vi "getViGetNextSample.vi"(8 "error in (no error)":errorcluster, 10 "name":string, 11 "LibReader in":refnum<class "LibReader.lvclass">) -> (0 "error out":errorcluster, 2 "pathViGetNextSample":path, 3 "LibReader out":refnum<class "LibReader.lvclass">)   [LabVIEW 2018, in "LibReader.lvclass"]
doc: "Get the path of get next sample vi."
uses:
  LibReader.lvclass
  LibReader.lvclass/LibReader.ctl
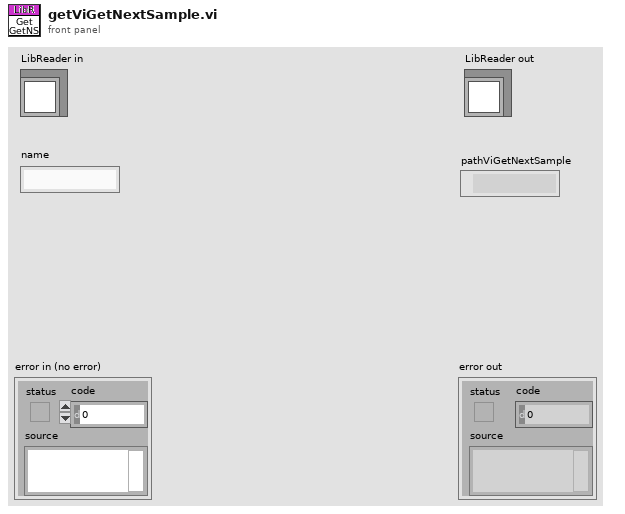
[diagram p1: front panel]
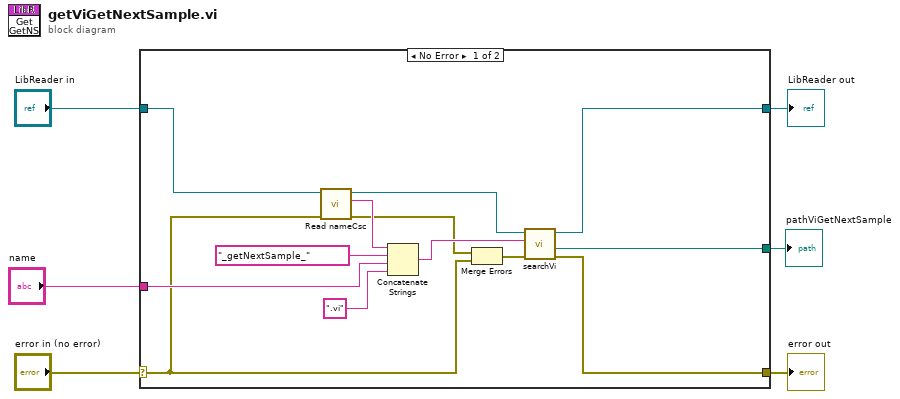
[diagram p0: block diagram]
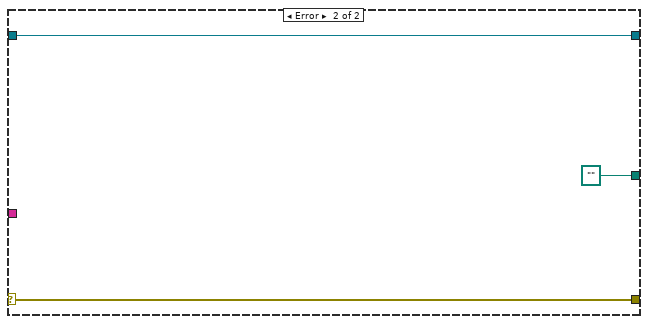
[diagram p2: hidden frame]
diagram:
  n1 = case shown="No Error" "error in (no error)" {
    selector: "error in (no error)" -> [w11 w22]
    tunnel: [w9 w22] -> w5
    tunnel: [w7 w21] -> w3
    tunnel: "LibReader in" -> [w14 w21]
    tunnel: [w19 path "" ("pathVi")] -> w2
    tunnel: "name" -> [w17 _]
    frame No Error {
      n2 = call "Read nameCsc.vi"("error in (no error)"=w11, "LibReader in"=w14) -> ("error out"=w12:errorcluster, "nameCsc"=w13:string, "LibReader out"=w8:refnum<class "LibReader.lvclass">)  [unwired: 7 in]
      n3 = Concatenate Strings(w13, "_getNextSample_" ("regExpr"), w17, ".vi" ("regExpr")) -> (w15:string)
      n4 = Merge Errors(w12, w11) -> (w10:errorcluster)
      n5 = call "searchVi.vi"("error in (no error)"=w10, "regExpr"=w15, "LibReader in"=w8) -> ("error out"=w9:errorcluster, "pathVi"=w19:path, "LibReader out"=w7:refnum<class "LibReader.lvclass">)  [unwired: 5 in, 1 out]
    }
    frame Error {
    }
  }
  "error out" <- w5
  "LibReader out" <- w3
  "pathViGetNextSample" <- w2
